vi "read_auto_file.vi"(0 "File Name With Extension":string) -> (1 "File Contents":string, 2 "file_status":string, 3 "error out":errorcluster)   [LabVIEW 2015]
uses:
  <vilib>/Rock Robotics/WPI/DriverStation/WPI_DriverStationStatusErrorCache.ctl
panel:
  out "lowercase file extension":string
  out "file or folder exists?":bool
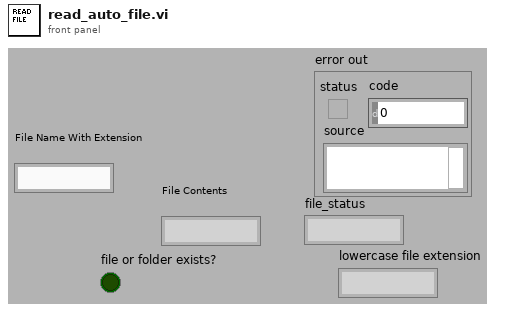
[diagram p1: front panel]
types:
  T1 = typedef "WPI_DriverStationStatusErrorCache.ctl" = enum16{"Get", "Set"}
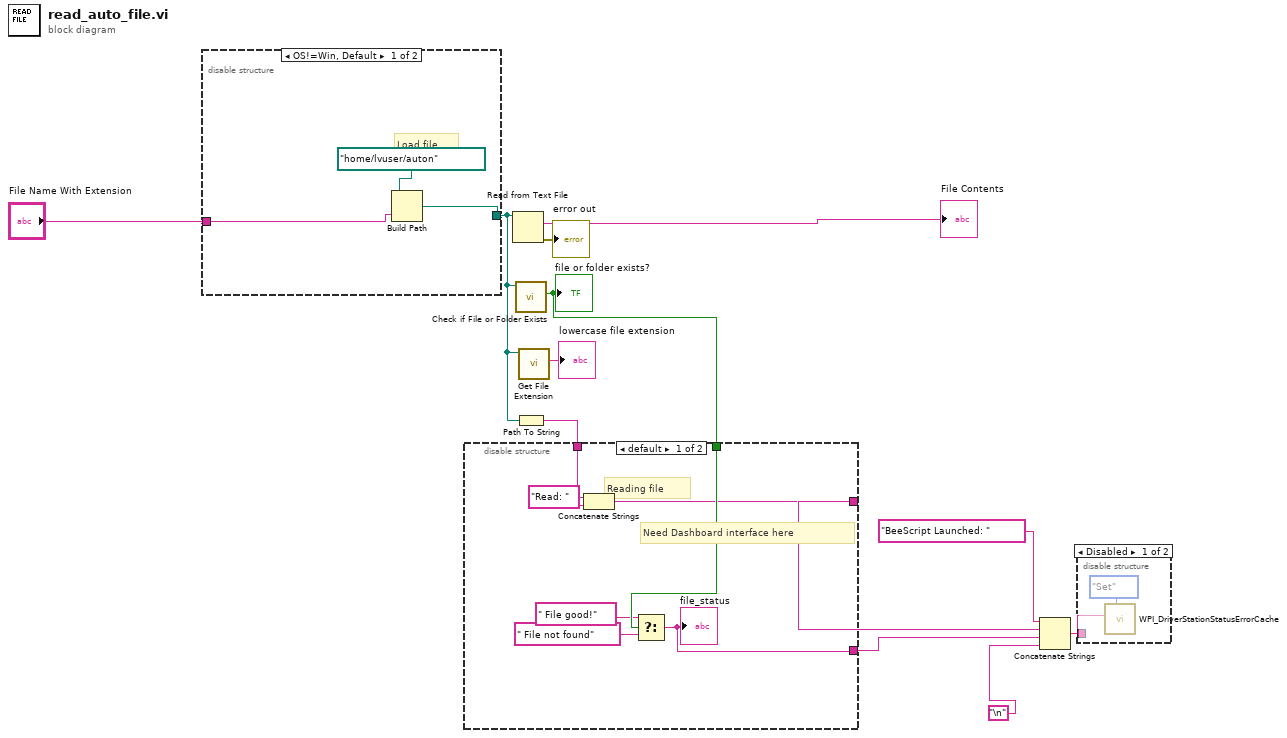
[diagram p0: block diagram]
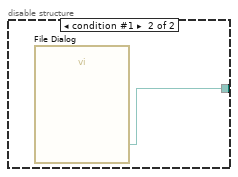
[diagram p4: hidden frame]
diagram:
  n1 = disable-structure shown="OS!=Win, Default" {
    disable-tunnel: "File Name With Extension" -> [w15 _]
    disable-tunnel: [w13 w16] -> w8
    frame condition #0 (active) {
      # "Load file"
      n2 = Build Path(base path=path "/home/lvuser/auton", name or relative path=w15) -> (appended path=w13:path)
    }
    frame condition #1 {
      n3 = call "File Dialog"() -> ("selected path"=w16:path)  [unwired: 7 in, 8 out]
    }
  }
  n4 = Read from Text File(file (use dialog)=w8) -> (text=→"File Contents":string, error out=→"error out":errorcluster)  [unwired: 1 in, 4 out]
  n5 = call <vilib>:"Check if File or Folder Exists.vi"("path"=w8) -> ("file or folder exists?"=w9:bool)  [unwired: 1 in, 9 out]
  "file or folder exists?" <- w9
  n6 = Path To String(path=w8) -> (string=w7:string)
  n7 = disable-structure shown="default" {
    disable-tunnel: w9 -> [w23 _]
    disable-tunnel: w7 -> [w19 _]
    disable-tunnel: [w18 _] -> w2
    disable-tunnel: [w17 _] -> w1
    frame condition #0 (active) {
      # "Need Dashboard interface here"
      # "Reading file"
      n8 = Concatenate Strings("Read: " ("string"), w19) -> (w18:string)
      n9 = Select(t=" File good!", s=w23, f=" File not found") -> (s? t:f=w17:string)
      "file_status" <- w17
    }
    frame condition #1 {
    }
  }
  n10 = call <vilib>:"Get File Extension.vi"("file"=w8) -> ("lowercase file extension"=→"lowercase file extension":string)  [unwired: 1 in, 9 out]
  n11 = Concatenate Strings("BeeScript Launched: " ("string"), w2, w1, "\n") -> (w5:string)
  n12 = disable-structure shown="Disabled" {
    disable-tunnel: w5 -> [w25 _]
    frame Disabled {
      n13 = call <vilib>:"WPI_DriverStationStatusErrorCache.vi"("StatusErrorCacheOp"=WPI_DriverStationStatusErrorCache."Set", "Error String"=w25) -> ()  [unwired: 1 in, 9 out]
    }
    frame Enabled {
    }
  }
